vi "Levels of Impulse Position.vi"() -> (0 "Size":i32)   [LabVIEW 2013]
uses:
  TD_Impulse Planes.ctl
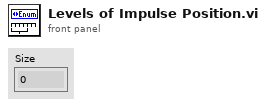
[diagram p1: front panel]
types:
  T1 = typedef "TD_Impulse Planes.ctl" = enum16{"Other", "Yaw", "Pitch", "Roll", "LARP", "RALP"}
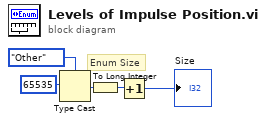
[diagram p0: block diagram]
diagram:
  # "Enum Size"
  n1 = Type Cast(type=TD_Impulse_Planes."Other" ("Impulse Plane"), x=u16 65535) -> (*(type *) &x=w3:T1)
  n2 = To Long Integer(number=w3) -> (32bit integer=w4:i32)
  n3 = Increment(x=w4) -> (x+1=→"Size":i32)
